vi "PCSLauncher.ProcCases.vi"(0 "i ref in":refnum<vi>, 1 "selector":string, 2 "Data":T1, 3 "call cluster":T2={"Object"="", "Selector"="", "CallType"=enum."synchronous", "Async Object"="", "Async Selector"="", "Data Descriptor"="", "Data"=[], "Error #"=0, "Expire"=0}, 5 "error in (no error)":errorcluster) -> (14 "i ref out":refnum<vi>, 17 "answer cluster":T2={"Object"="", "Selector"="", "CallType"=enum."synchronous", "Async Object"="", "Async Selector"="", "Data Descriptor"="", "Data"=[], "Error #"=0, "Expire"=0}, 19 "error out":errorcluster)   [LabVIEW 2014, in "PCSLauncher.lvlib"]
doc: "This method is called by a process from within the default case in the event loop. The methods of a class that are linked to events will be called from THIS method. Add your code here."
uses:
  PCSLauncher.lvlib
  CS_Core/CSSystem/CoreDefs/CoreDefs.call_type.ctl
  CS_Core/BaseProcess/BaseProcess.descriptor string definition.ctl
  CS_Core/CSSystem/CoreDefs/CoreDefs.rawDataType.ctl
  CS_Core/CSSystem/CSSystemLib/CSSystemLib.object condition.ctl
  CS_Core/CSSystem/CoreLib/CoreLib.string 2 byte array.vi
  CS_Core/CSSystem/CoreLib/CoreLib.lvlib
  CS_Core/BaseProcess/BaseProcess.lvlib
  CS_Core/CSSystem/CSSystemLib/CSSystemLib.lvlib
  CS_Core/CAEObj/CAEObj.lvlib
  PH_Basics/PH_Common/PH_Common.lvlib
  PH_Basics/PH_Class/PH_Class.lvlib
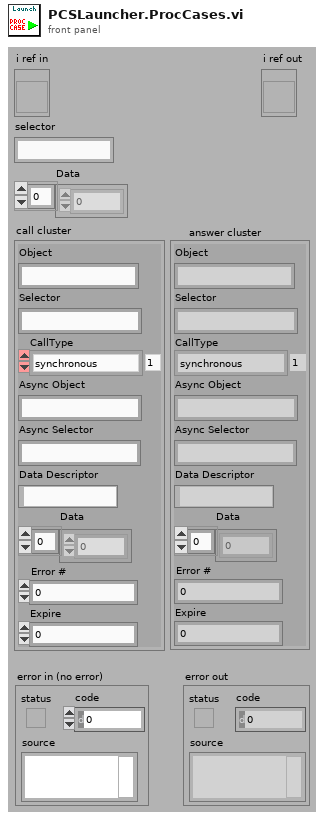
[diagram p1: front panel]
types:
  T1 = typedef "CoreDefs.rawDataType.ctl" = i8[]
  T2 = typedef "CoreDefs.call_type.ctl" = cluster{"Object":string, "Selector":string, "CallType":enum16{"simple", "synchronous", "asynchronous"}, "Async Object":string, "Async Selector":string, "Data Descriptor":T3, "Data":T1, "Error #":i32, "Expire":u32}
  T3 = typedef "BaseProcess.lvlib/BaseProcess.descriptor string definition.ctl" = string
  T4 = typedef "CSSystemLib.lvlib/CSSystemLib.object condition.ctl" = i32
  T5 = typedef "PCSLauncher.lvlib/PCSLauncher.i attribute.ctl" = cluster{"PCS Systems":cluster{"GUI Ref":refnum<vi>, "Super alive?":bool, "Start-GOG alive?":bool}[], "GUI Refs":cluster{"Delete":refnum<vi>, "Launch PCS":refnum<vi>}}
  T6 = cluster{"GUI Ref":refnum<vi>, "Super alive?":bool, "Start-GOG alive?":bool}[]
  T7 = cluster{"GUI Ref":refnum<vi>, "Super alive?":bool, "Start-GOG alive?":bool}
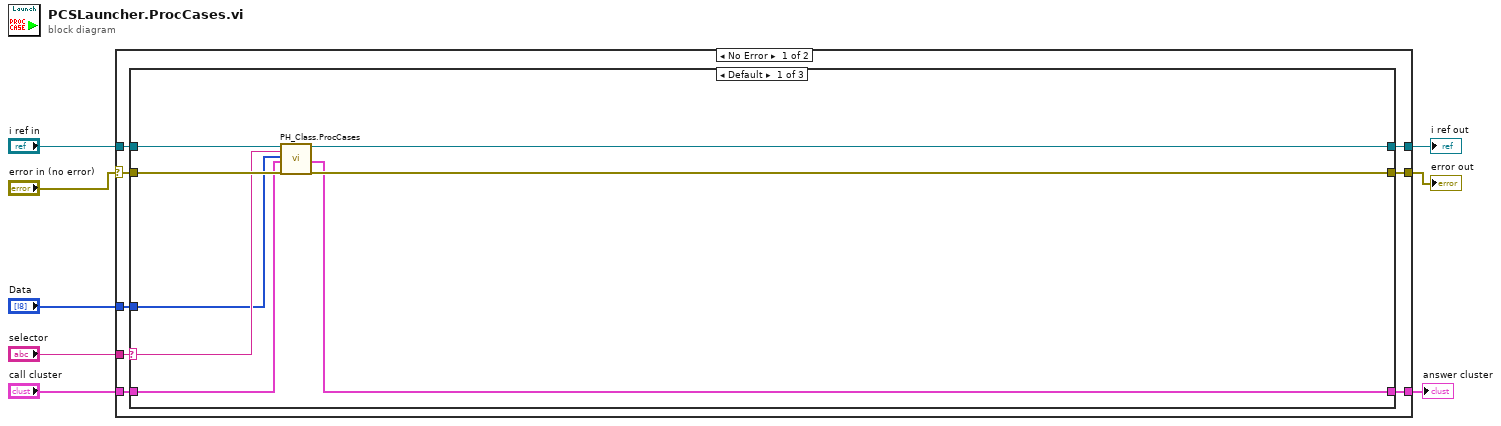
[diagram p0: block diagram]
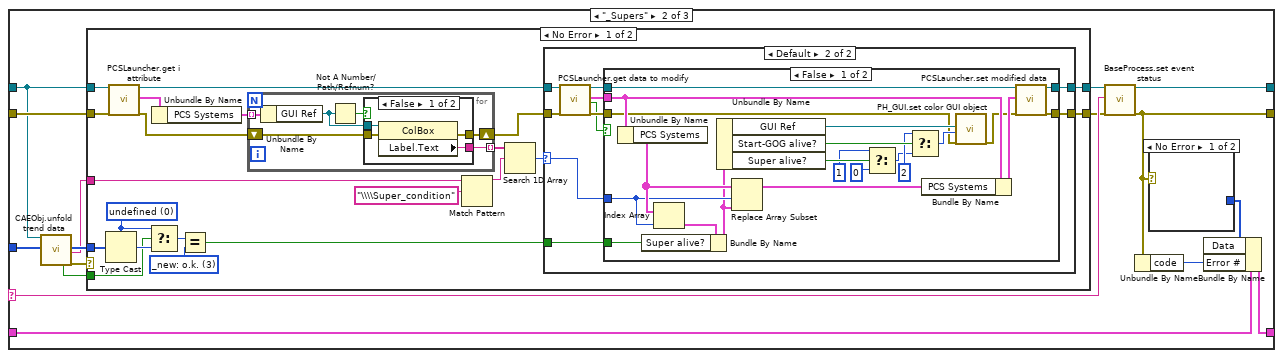
[diagram p2: hidden frame]
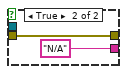
[diagram p5: hidden frame]
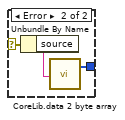
[diagram p7: hidden frame]
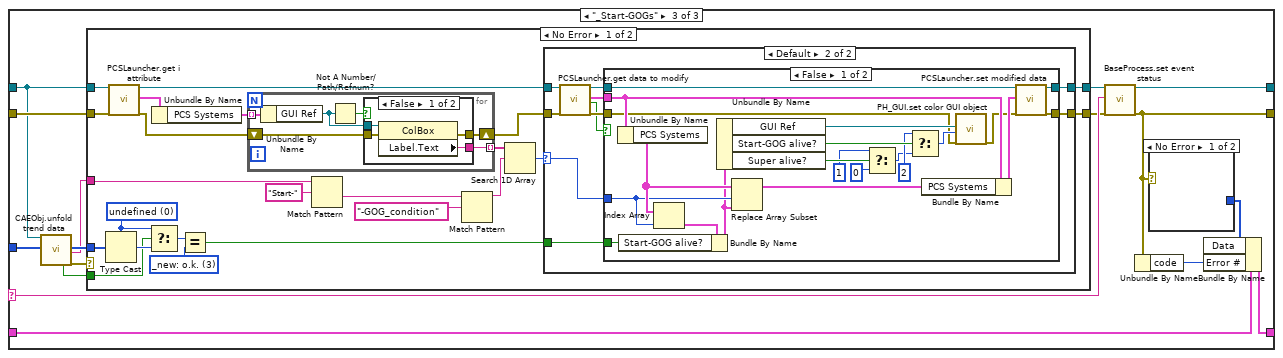
[diagram p8: hidden frame]
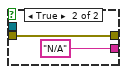
[diagram p11: hidden frame]
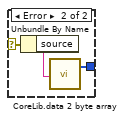
[diagram p13: hidden frame]
diagram:
  n1 = case shown="No Error" "error in (no error)" {
    selector: "error in (no error)" -> [w9 w206]
    tunnel: "selector" -> [w16 _]
    tunnel: [w15 w205] -> w7
    tunnel: "call cluster" -> [w14 w205]
    tunnel: "i ref in" -> [w13 w207]
    tunnel: [w12 w207] -> w4
    tunnel: [w11 w206] -> w3
    tunnel: "Data" -> [w10 _]
    frame No Error {
      n2 = case shown="Default" w16 {
        selector: w16 -> [w19 w36 w125]
        tunnel: w10 -> [w17 w26 w115]
        tunnel: w13 -> [w18 w25 w114]
        tunnel: [w24 w38 w127] -> w12
        tunnel: w14 -> [w20 w35 w124]
        tunnel: [w21 w34 w123] -> w15
        tunnel: w9 -> [w23 w29 w118]
        tunnel: [w22 w37 w126] -> w11
        frame Default {
          n3 = call "PH_Class.ProcCases.vi"("i ref in"=w18, "selector"=w19, "Data"=w17, "call cluster"=w20, "error in (no error)"=w23) -> ("i ref out"=w24:refnum<vi>, "answer cluster"=w21:T2, "error out"=w22:errorcluster)  [unwired: 12 in]
        }
        frame "_Supers" {
          n4 = call "CAEObj.unfold trend data.vi"("i ref in"=w25, "raw trend data"=w26) -> ("no link"=w32:bool, "data"=w31:i8[], "serviceName"=w30:string, "error out"=w33:errorcluster)  [unwired: 9 in, 5 out]
          n5 = case shown="No Error" w33 {
            tunnel: [w44 w110] -> w28
            tunnel: w25 -> [w41 w110]
            tunnel: w29 -> [w59 w109]
            tunnel: w31 -> [w58 _]
            tunnel: w32 -> [w52 _]
            tunnel: w30 -> [w54 _]
            tunnel: [w43 w109] -> w27
            frame No Error {
              w56 = T4 3 items=["undefined", "executing constructor", "_new: error", "_new: o.k.", "executing destructor"] ("x")
              w60 = T4 0 items=["undefined", "executing constructor", "_new: error", "_new: o.k.", "executing destructor"] ("condition")
              n6 = Type Cast(type=w60, x=w58) -> (*(type *) &x=w61:T4)
              n7 = call "PCSLauncher.get i attribute.vi"("i ref in"=w41, "error in (no error)"=w59) -> ("i ref out"=w46:refnum<vi>, "i attribute"=w55:T5, "error out"=w50:errorcluster)  [unwired: 15 in]
              n8 = Select(t=w60, s=w52, f=w61) -> (s? t:f=w57:T4)
              n9 = Unbundle By Name(w55) -> ("PCS Systems"=w51:T6)
              n10 = Equal?(x=w57, y=w56) -> (x = y?=w42:bool)
              n11 = for {
                tunnel: [w102] -> w49 mode=indexing
                shift-right: [w101] -> w45
                shift-left: w50 -> [w100]
                tunnel: w51 -> [w98] mode=indexing
                n12 = Unbundle By Name(w98) -> ("GUI Ref"=w97:refnum<vi>)
                n13 = Not A Number/Path/Refnum?(number/path/refnum=w97) -> (NaN/Path/Refnum?=w99:bool)
                n14 = case shown="False" w99 {
                  tunnel: w97 -> [w106 _]
                  tunnel: [w103 "N/A" ("Label.Text")] -> w102
                  tunnel: [w105 w107] -> w101
                  tunnel: w100 -> [w104 w107]
                  frame False {
                    n15 = property class="ColBox"(reference=w106, error in=w104) -> (error out=w105:errorcluster, "Label.Text"=w103:string)  [unwired: 1 out]
                  }
                  frame True {
                  }
                }
              }
              n16 = Match Pattern(string=w54, regular expression="\\\\Super_condition") -> (before substring=w47:string)  [unwired: 1 in, 3 out]
              n17 = Search 1D Array(1D array=w49, element=w47) -> (index of element=w48:i32)  [unwired: 1 in]
              n18 = case shown="Default" w48 {
                selector: w48 -> [_ w65]
                tunnel: w46 -> [w63 w73]
                tunnel: w45 -> [w62 w72]
                tunnel: [w63 w70] -> w44
                tunnel: [w62 w68] -> w43
                tunnel: w42 -> [_ w64]
                frame -1 {
                }
                frame Default {
                  n19 = call "PCSLauncher.get data to modify.vi"("i ref in"=w73, "error in (no error)"=w72) -> ("i ref out"=w71:refnum<vi>, "i attribute"=w67:T5, "timed out"=w66:bool, "error out"=w69:errorcluster)  [unwired: 14 in]
                  n20 = case shown="False" w66 {
                    tunnel: w71 -> [w94 w96]
                    tunnel: [w93 w96] -> w70
                    tunnel: w69 -> [w75 w95]
                    tunnel: [w92 w95] -> w68
                    tunnel: w67 -> [w90 _]
                    tunnel: w65 -> [w88 _]
                    tunnel: w64 -> [w85 _]
                    frame False {
                      n21 = Unbundle By Name(w90) -> ("PCS Systems"=w89:T6)
                      n22 = Index Array(array=w89, index=w88) -> (element=w86:T7)
                      n23 = Bundle By Name(cluster=w86, "Super alive?"=w85) -> (w84:T7)
                      n24 = Unbundle By Name(w84) -> ("GUI Ref"=w83:refnum<vi>, "Start-GOG alive?"=w82:bool, "Super alive?"=w79:bool)
                      n25 = Replace Array Subset(array=w89, new element=w84, index=w88) -> (w87:T6)
                      n26 = Select(t=1 ("State"), s=w79, f=0) -> (s? t:f=w78:i32)
                      n27 = Select(t=2 ("State"), s=w82, f=w78) -> (s? t:f=w80:i32)
                      n28 = Bundle By Name(cluster=w90, "PCS Systems"=w87) -> (w91:T5)
                      n29 = call "PH_GUI.set color GUI object.vi"("GUI object Ref"=w83, "State"=w80, "error in (no error)"=w75) -> ("error out"=w74:errorcluster)  [unwired: 16 in]
                      n30 = call "PCSLauncher.set modified data.vi"("i ref in"=w94, "i attribute"=w91, "error in (no error)"=w74) -> ("i ref out"=w93:refnum<vi>, "error out"=w92:errorcluster)  [unwired: 15 in]
                    }
                    frame True {
                    }
                  }
                }
              }
            }
            frame Error {
            }
          }
          n31 = call "BaseProcess.set event status.vi"("i ref in"=w28, "EventStatus"=w36, "error in (no error)"=w27) -> ("i ref out"=w38:refnum<vi>, "error out"=w37:errorcluster)  [unwired: 14 in, 1 out]
          n32 = Unbundle By Name(w37) -> ("code"=w40:i32)
          n33 = case shown="No Error" w37 {
            selector: w37 -> [_ w113]
            tunnel: [_ w111] -> w39
            frame No Error {
            }
            frame Error {
              n34 = Unbundle By Name(w113) -> ("source"=w112:string)
              n35 = call-poly "CoreLib.data 2 byte array.vi"("string"=w112) -> ("byteArray out"=w111:T1)  [unwired: 18 in]
            }
          }
          n36 = Bundle By Name(cluster=w35, "Data"=w39, "Error #"=w40) -> (w34:T2)
        }
        frame "_Start-GOGs" {
          n37 = call "CAEObj.unfold trend data.vi"("i ref in"=w114, "raw trend data"=w115) -> ("no link"=w121:bool, "data"=w120:i8[], "serviceName"=w119:string, "error out"=w122:errorcluster)  [unwired: 9 in, 5 out]
          n38 = case shown="No Error" w122 {
            tunnel: [w135 w201] -> w117
            tunnel: w114 -> [w150 w201]
            tunnel: w118 -> [w149 w200]
            tunnel: w120 -> [w148 _]
            tunnel: w121 -> [w143 _]
            tunnel: w119 -> [w131 _]
            tunnel: [w134 w200] -> w116
            frame No Error {
              w146 = T4 3 items=["undefined", "executing constructor", "_new: error", "_new: o.k.", "executing destructor"] ("x")
              w151 = T4 0 items=["undefined", "executing constructor", "_new: error", "_new: o.k.", "executing destructor"] ("condition")
              n39 = Type Cast(type=w151, x=w148) -> (*(type *) &x=w152:T4)
              n40 = call "PCSLauncher.get i attribute.vi"("i ref in"=w150, "error in (no error)"=w149) -> ("i ref out"=w137:refnum<vi>, "i attribute"=w145:T5, "error out"=w141:errorcluster)  [unwired: 15 in]
              n41 = Select(t=w151, s=w143, f=w152) -> (s? t:f=w147:T4)
              n42 = Unbundle By Name(w145) -> ("PCS Systems"=w142:T6)
              n43 = Equal?(x=w147, y=w146) -> (x = y?=w133:bool)
              n44 = for {
                tunnel: [w193] -> w140 mode=indexing
                shift-right: [w192] -> w136
                shift-left: w141 -> [w191]
                tunnel: w142 -> [w189] mode=indexing
                n45 = Unbundle By Name(w189) -> ("GUI Ref"=w188:refnum<vi>)
                n46 = Not A Number/Path/Refnum?(number/path/refnum=w188) -> (NaN/Path/Refnum?=w190:bool)
                n47 = case shown="False" w190 {
                  tunnel: w188 -> [w197 _]
                  tunnel: [w194 "N/A" ("Label.Text")] -> w193
                  tunnel: [w196 w198] -> w192
                  tunnel: w191 -> [w195 w198]
                  frame False {
                    n48 = property class="ColBox"(reference=w197, error in=w195) -> (error out=w196:errorcluster, "Label.Text"=w194:string)  [unwired: 1 out]
                  }
                  frame True {
                  }
                }
              }
              n49 = Match Pattern(string=w131, regular expression="Start-") -> (after substring=w130:string)  [unwired: 1 in, 3 out]
              n50 = Match Pattern(string=w130, regular expression="-GOG_condition") -> (before substring=w138:string)  [unwired: 1 in, 3 out]
              n51 = Search 1D Array(1D array=w140, element=w138) -> (index of element=w139:i32)  [unwired: 1 in]
              n52 = case shown="Default" w139 {
                selector: w139 -> [_ w156]
                tunnel: w137 -> [w154 w164]
                tunnel: w136 -> [w153 w163]
                tunnel: [w154 w161] -> w135
                tunnel: [w153 w159] -> w134
                tunnel: w133 -> [_ w155]
                frame -1 {
                }
                frame Default {
                  n53 = call "PCSLauncher.get data to modify.vi"("i ref in"=w164, "error in (no error)"=w163) -> ("i ref out"=w162:refnum<vi>, "i attribute"=w158:T5, "timed out"=w157:bool, "error out"=w160:errorcluster)  [unwired: 14 in]
                  n54 = case shown="False" w157 {
                    tunnel: w162 -> [w185 w187]
                    tunnel: [w184 w187] -> w161
                    tunnel: w160 -> [w166 w186]
                    tunnel: [w183 w186] -> w159
                    tunnel: w158 -> [w181 _]
                    tunnel: w156 -> [w179 _]
                    tunnel: w155 -> [w176 _]
                    frame False {
                      n55 = Unbundle By Name(w181) -> ("PCS Systems"=w180:T6)
                      n56 = Index Array(array=w180, index=w179) -> (element=w177:T7)
                      n57 = Bundle By Name(cluster=w177, "Start-GOG alive?"=w176) -> (w175:T7)
                      n58 = Unbundle By Name(w175) -> ("GUI Ref"=w174:refnum<vi>, "Start-GOG alive?"=w173:bool, "Super alive?"=w170:bool)
                      n59 = Replace Array Subset(array=w180, new element=w175, index=w179) -> (w178:T6)
                      n60 = Select(t=1 ("State"), s=w170, f=0) -> (s? t:f=w169:i32)
                      n61 = Select(t=2 ("State"), s=w173, f=w169) -> (s? t:f=w171:i32)
                      n62 = Bundle By Name(cluster=w181, "PCS Systems"=w178) -> (w182:T5)
                      n63 = call "PH_GUI.set color GUI object.vi"("GUI object Ref"=w174, "State"=w171, "error in (no error)"=w166) -> ("error out"=w165:errorcluster)  [unwired: 16 in]
                      n64 = call "PCSLauncher.set modified data.vi"("i ref in"=w185, "i attribute"=w182, "error in (no error)"=w165) -> ("i ref out"=w184:refnum<vi>, "error out"=w183:errorcluster)  [unwired: 15 in]
                    }
                    frame True {
                    }
                  }
                }
              }
            }
            frame Error {
            }
          }
          n65 = call "BaseProcess.set event status.vi"("i ref in"=w117, "EventStatus"=w125, "error in (no error)"=w116) -> ("i ref out"=w127:refnum<vi>, "error out"=w126:errorcluster)  [unwired: 14 in, 1 out]
          n66 = Unbundle By Name(w126) -> ("code"=w129:i32)
          n67 = case shown="No Error" w126 {
            selector: w126 -> [_ w204]
            tunnel: [_ w202] -> w128
            frame No Error {
            }
            frame Error {
              n68 = Unbundle By Name(w204) -> ("source"=w203:string)
              n69 = call-poly "CoreLib.data 2 byte array.vi"("string"=w203) -> ("byteArray out"=w202:T1)  [unwired: 18 in]
            }
          }
          n70 = Bundle By Name(cluster=w124, "Data"=w128, "Error #"=w129) -> (w123:T2)
        }
      }
    }
    frame Error {
    }
  }
  "answer cluster" <- w7
  "i ref out" <- w4
  "error out" <- w3
